vi "Shutdown Core.vi"(8 "error in (no error)":errorcluster, 11 "Test Consumer in":refnum<class "Test UI Consumer.lvclass">) -> (0 "error out":errorcluster, 3 "Test Consumer out":refnum<class "Test UI Consumer.lvclass">)   [LabVIEW 2027, in "Test UI Consumer.lvclass"]
uses:
  Test UI Consumer.lvclass
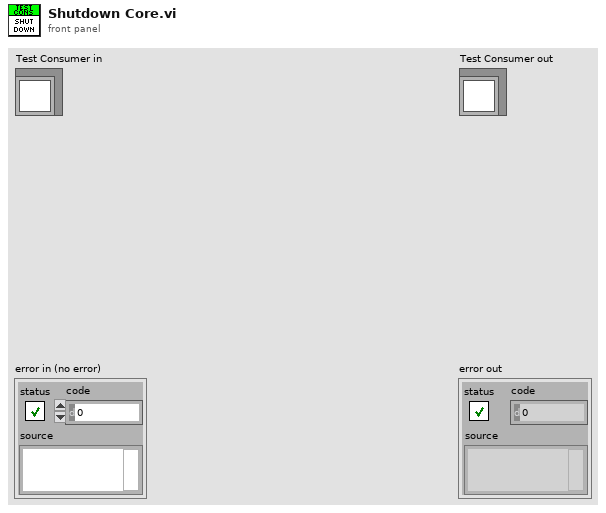
[diagram p1: front panel]
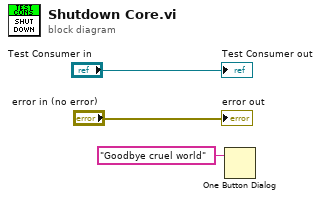
[diagram p0: block diagram]
diagram:
  n1 = One Button Dialog(message="Goodbye cruel world") -> ()  [unwired: 1 in, 1 out]
  "error out" <- "error in (no error)"
  "Test Consumer out" <- "Test Consumer in"
